vi "Required LV Version.vi"(8 "error in (no error)":errorcluster, 11 "Caraya Item in":refnum<class "Caraya Item.lvclass">) -> (0 "error out":errorcluster, 1 "64 Bit?":bool, 2 "LV Year":u32)   [LabVIEW 2019, in "Caraya Library.lvlib" / "Caraya Item.lvclass"]
uses:
  Caraya Item.lvclass
  Caraya Item.lvclass/Caraya Item.ctl
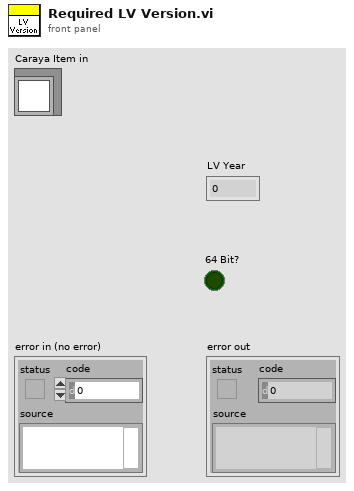
[diagram p1: front panel]
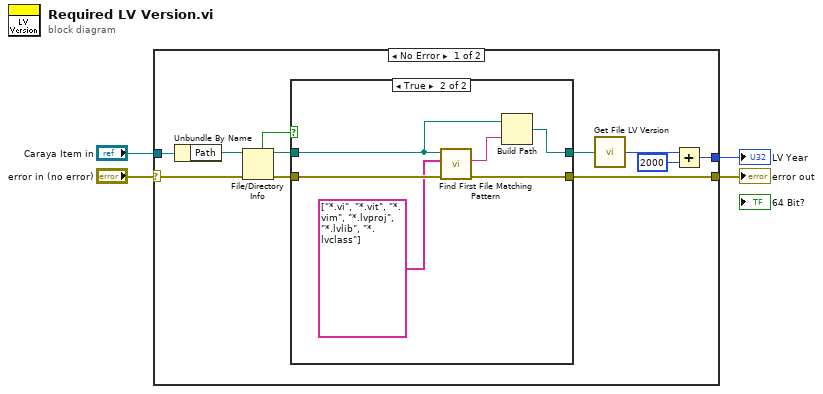
[diagram p0: block diagram]
diagram:
  n1 = case shown="No Error" "error in (no error)" {
    selector: "error in (no error)" -> [w12 w24]
    tunnel: "Caraya Item in" -> [w15 _]
    tunnel: [w14 w24] -> w3
    tunnel: [w6 _] -> w2
    frame No Error {
      n2 = Unbundle By Name(w15) -> ("Path"=w9:path)
      n3 = File/Directory Info(path=w9, error in=w12) -> (path out=w10:path, directory=w13:bool, error out=w11:errorcluster)  [unwired: 4 out]
      n4 = case shown="True" w13 {
        tunnel: [w17 w22] -> w14
        tunnel: w11 -> [w17 w23]
        tunnel: w10 -> [w16 w20]
        tunnel: [w16 w18] -> w8
        frame False {
        }
        frame True {
          n5 = call "Find First File Matching Pattern.vi"("error in (no error)"=w23, "Patterns"=string[] ["*.vi", "*.vit", "*.vim", "*.lvproj", "*.lvlib", "*.lvclass"], "Path"=w20) -> ("error out"=w22:errorcluster, "Filename"=w19:string)  [unwired: 7 in]
          n6 = Build Path(base path=w20, name or relative path=w19) -> (appended path=w18:path)
        }
      }
      n7 = call "Get File LV Version.vi"("Path"=w8) -> ("LV Version"=w7:u32)  [unwired: 1 in]
      n8 = Add(x=w7, y=u32 2000) -> (x+y=w6:u32)
    }
    frame Error {
    }
  }
  "error out" <- w3
  "LV Year" <- w2
